vi "TC Loop.vi"(9 "Period (us)":u32=1000, 10 "Iterations":i32=1000, 11 "Pre-allocated Timestamp Array":u64[](array[numeric])) -> (3 "Timestamp Array":u64[](array[numeric]))   [LabVIEW 2014]
uses:
  Instance           1 15Saved   TC Loop .vi
  <vilib>/NI_Real-Time Target Support.lvlib
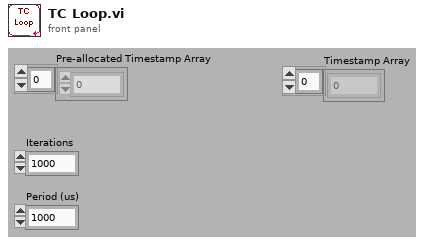
[diagram p1: front panel]
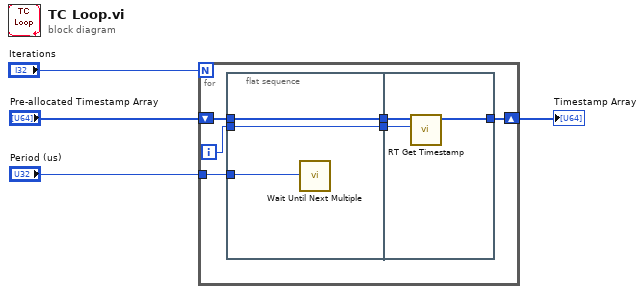
[diagram p0: block diagram]
diagram:
  n1 = for {
    N: "Iterations" -> [_]
    shift-right: [w10] -> w1
    shift-left: "Pre-allocated Timestamp Array" -> [w9]
    tunnel: "Period (us)" -> [w5]
    i -> [w8]
    n2 = flat-sequence {
      tunnel: w9 -> [w13]
      tunnel: [w13] -> w7
      tunnel: w8 -> [w12]
      tunnel: [w12] -> w6
      tunnel: w5 -> [w11]
      tunnel: w7 -> [w15]
      tunnel: w6 -> [w14]
      tunnel: [w16] -> w10
      frame #0 {
        n3 = call "Wait Until Next Multiple"("Count(uSec)"=w11) -> ()  [unwired: 1 out]
      }
      frame #1 {
        n4 = call <vilib>:"RT Get Timestamp.vi"("iteration"=w14, "timestamp array in"=w15) -> ("timestamp array out"=w16:u64[])  [unwired: 8 in, 1 out]
      }
    }
  }
  "Timestamp Array" <- w1
